vi "Configure Standard Waveform.vi"(8 "error in (no error)":errorcluster, 10 "Std Waveform Setting":T1={"Waveform Function (1: Sine)"=1, "Frequency (1000 Hz)"=1000.0, "Amplitude (1)"=1.0, "Unit (0: Vpp)"=0, "DC Offset (0.00 V)"=0.0} {"Unit (0: Vpp)" items=["Vpp", "Vrms", "dB"]; "Waveform Function (1: Sine)" items=["DC", "Sine", "Square", "Triangle", "Ramp", "Pulse", "Noise", "Sinc", "Negative Ramp", "Exponential Rise", "Exponential Fall", "Cardiac"]}, 11 "Agilent 33210A in":refnum<class "Agilent 33210A.lvclass">) -> (0 "error out":errorcluster, 3 "Agilent 33210A out":refnum<class "Agilent 33210A.lvclass">)   [LabVIEW 2023, in "Func Generator.lvlib" / "Agilent 33210A.lvclass"]
uses:
  Agilent 33210A.lvclass
  Agilent 33210A.lvclass/Agilent 33210A.ctl
  <instrlib>/Agilent 33XXX Series/Agilent 33XXX Series.lvlib
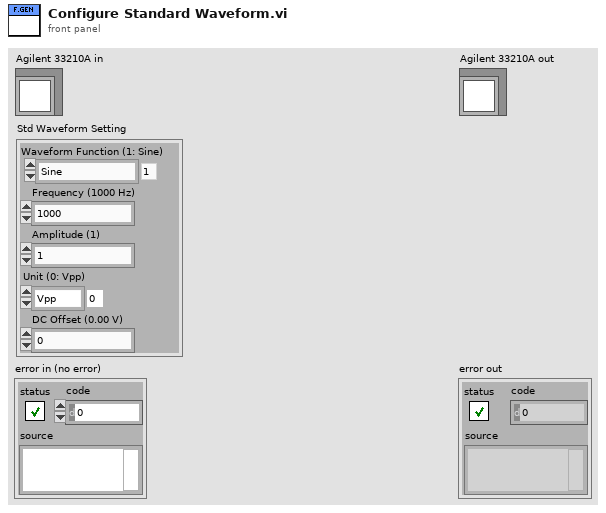
[diagram p1: front panel]
types:
  T1 = cluster{"Waveform Function (1: Sine)":u16, "Frequency (1000 Hz)":dbl, "Amplitude (1)":dbl, "Unit (0: Vpp)":u16, "DC Offset (0.00 V)":dbl}
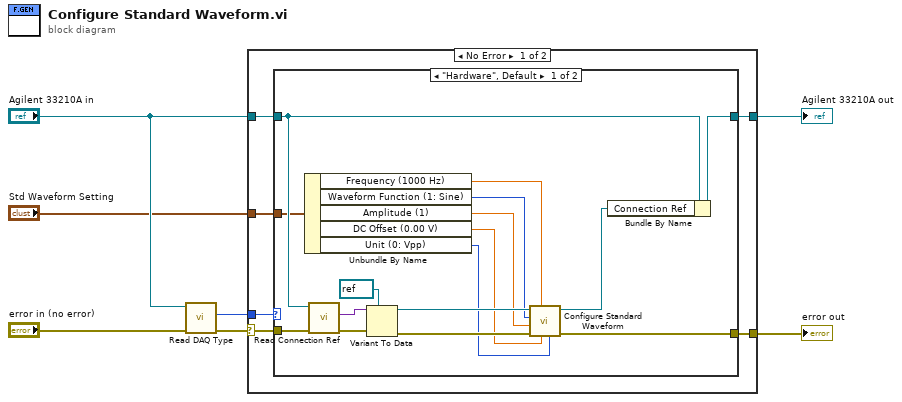
[diagram p0: block diagram]
diagram:
  n1 = call-dynamic "Read DAQ Type.vi"("error in (no error)"="error in (no error)", "Agilent 33210A in"="Agilent 33210A in") -> ("error out"=w6:errorcluster, "DAQ Type"=w5:enum16{"Hardware", "Simulation"})  [unwired: 7 in, 1 out]
  n2 = case shown="No Error" w6 {
    selector: w6 -> [w13 w32]
    tunnel: w5 -> [w12 _]
    tunnel: "Agilent 33210A in" -> [w11 w33]
    tunnel: [w10 w33] -> w3
    tunnel: "Std Waveform Setting" -> [w9 _]
    tunnel: [w8 w32] -> w1
    frame No Error {
      n3 = case shown="\"Hardware\", Default" w12 {
        tunnel: w13 -> [w29 w30]
        tunnel: w11 -> [w24 w31]
        tunnel: [w23 w31] -> w10
        tunnel: w9 -> [w20 _]
        tunnel: [w14 w30] -> w8
        frame "Hardware", Default {
          n4 = Unbundle By Name(w20) -> ("Frequency (1000 Hz)"=w19:dbl, "Waveform Function (1: Sine)"=w18:u16, "Amplitude (1)"=w17:dbl, "DC Offset (0.00 V)"=w16:dbl, "Unit (0: Vpp)"=w15:u16)
          n5 = call-dynamic "Read Connection Ref.vi"("error in (no error)"=w29, "Agilent 33210A in"=w24) -> ("error out"=w28:errorcluster, "Connection Ref"=w27:variant)  [unwired: 7 in, 1 out]
          n6 = Variant To Data(error in=w28, type=refnum<visa-resource-name> refnum ("VISA resource name"), Variant=w27) -> (data=w21:refnum<visa-resource-name>, error out=w25:errorcluster)
          n7 = call <instrlib>:"Configure Standard Waveform.vi"("Unit (0: Vpp)"=w15, "DC Offset (0.00 V)"=w16, "Frequency (1000 Hz)"=w19, "error in (no error)"=w25, "Amplitude (1)"=w17, "Waveform Function (1: Sine)"=w18, "VISA resource name"=w21) -> ("error out"=w14:errorcluster, "VISA resource name out"=w22:refnum<visa-resource-name>)  [unwired: 3 in]
          n8 = Bundle By Name(cluster=w24, "Connection Ref"=w22) -> (w23:refnum<class "Agilent 33210A.lvclass">)
        }
        frame "Simulation" {
        }
      }
    }
    frame Error {
    }
  }
  "error out" <- w1
  "Agilent 33210A out" <- w3
